vi "graph_xy.vi"() -> ()   [LabVIEW 2012]
panel:
  out "y = 2x+1 Graph":cluster{i32, i32}[](graph)
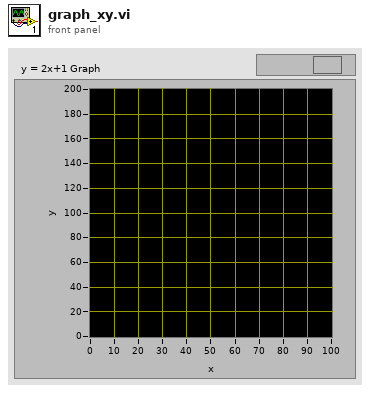
[diagram p1: front panel]
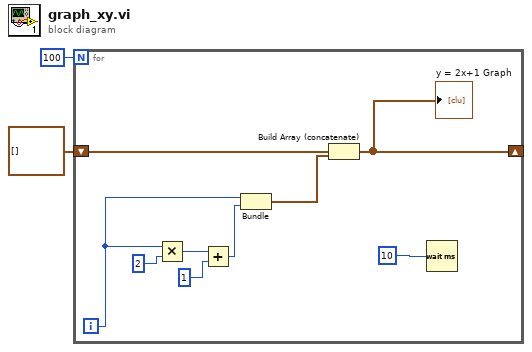
[diagram p0: block diagram]
diagram:
  n1 = for {
    N: 100 -> [_]
    shift-right: [w4] -> _
    shift-left: cluster{i32, i32}[] [] -> [w3]
    i -> [w7]
    n2 = Multiply(x=w7, y=2) -> (x*y=w9:i32)
    n3 = Add(x=w9, y=1) -> (x+y=w6:i32)
    n4 = Bundle(w7, w6) -> (w5:cluster{i32, i32})  [unwired: 1 in]
    n5 = Build Array (concatenate)(w3, w5) -> (w4:cluster{i32, i32}[])
    "y = 2x+1 Graph" <- w4
    n6 = Wait (ms)(milliseconds to wait=10) -> ()  [unwired: 1 out]
  }
